vi "Read Shared Variables - SuNLaMP 9216 Slot 3.vi"(9 "channel errors in (no errors)":errorcluster[](array[cluster])) -> (1 "channel errors out":errorcluster[](array[cluster]), 2 "data":dbl[](array[numeric]), 3 "UUIDs":string[](array[string])=["Flow Rate [g/s]", "Density [g/cm^3]", "Return Filter dP [psid]", "Outlet Filter and Flowmeter dp [psid]", "Cooler dP [psid]", "Cooler CO2 In [F]", "Cooler CO2 Out [F]", "Pump Frequency [%]", "Recirc Valve Open [%]"])   [LabVIEW 2020]
uses:
  <vilib>/Utility/error.llb/Error Cluster From Error Code.vi
  <vilib>/ErrorRing/Error Ring.xnode
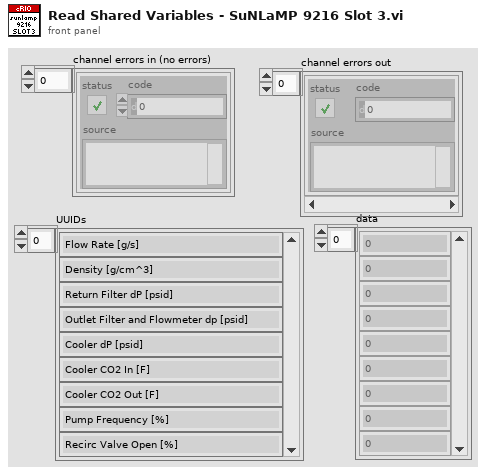
[diagram p1: front panel]
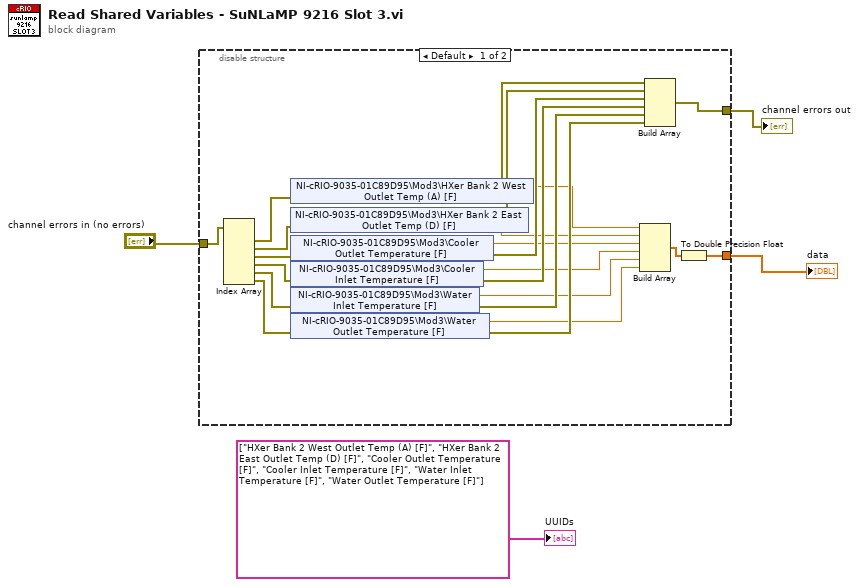
[diagram p0: block diagram]
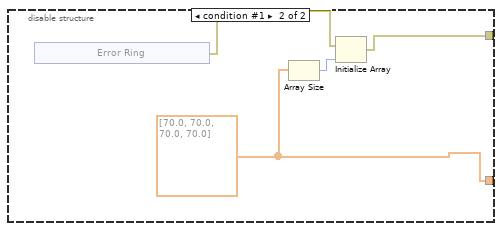
[diagram p2: hidden frame]
diagram:
  n1 = disable-structure shown="Default" {
    disable-tunnel: [w18 w28] -> w3
    disable-tunnel: "channel errors in (no errors)" -> [w17 _]
    disable-tunnel: [w12 w29] -> w1
    frame condition #0 (active) {
      n2 = Index Array(array=w17) -> (element #1=w9:errorcluster, element #2=w10:errorcluster, element #3=w16:errorcluster, element #4=w15:errorcluster, element #5=w14:errorcluster, element #6=w13:errorcluster)  [unwired: 6 in]
      n3 = shared-variable "NI-cRIO-9035-01C89D95\\Mod3\\HXer Bank 2 West Outlet Temp (A) [F]"(error in=w9) -> (w5:dbl, error out=w8:errorcluster)
      n4 = shared-variable "NI-cRIO-9035-01C89D95\\Mod3\\HXer Bank 2 East Outlet Temp (D) [F]"(error in=w10) -> (w6:dbl, error out=w7:errorcluster)
      n5 = shared-variable "NI-cRIO-9035-01C89D95\\Mod3\\Cooler Outlet Temperature [F]"(error in=w16) -> (w19:dbl, error out=w23:errorcluster)
      n6 = shared-variable "NI-cRIO-9035-01C89D95\\Mod3\\Cooler Inlet Temperature [F]"(error in=w15) -> (w20:dbl, error out=w24:errorcluster)
      n7 = shared-variable "NI-cRIO-9035-01C89D95\\Mod3\\Water Inlet Temperature [F]"(error in=w14) -> (w21:dbl, error out=w25:errorcluster)
      n8 = shared-variable "NI-cRIO-9035-01C89D95\\Mod3\\Water Outlet Temperature [F]"(error in=w13) -> (w22:dbl, error out=w26:errorcluster)
      n9 = Build Array(w5, w6, w19, w20, w21, w22) -> (w11:dbl[])
      n10 = Build Array(w8, w7, w23, w24, w25, w26) -> (w18:errorcluster[])
      n11 = To Double Precision Float(number=w11) -> (double precision float=w12:dbl[])
    }
    frame condition #1 {
      w29 = dbl[] [70.0, 70.0, 70.0, 70.0] ("data")
      n12 = xnode "Error Ring"() -> ("error out"=w27:errorcluster)
      n13 = Array Size(array=w29) -> (size(s)=w30:i32)
      n14 = Initialize Array(w27, w30) -> (w28:errorcluster[])
    }
  }
  "data" <- w1
  "channel errors out" <- w3
  "UUIDs" <- string[] ["HXer Bank 2 West Outlet Temp (A) [F]", "HXer Bank 2 East Outlet Temp (D) [F]", "Cooler Outlet Temperature [F]", "Cooler Inlet Temperature [F]", "Water Inlet Temperature [F]", "Water Outlet Temperature [F]"]
